vi "GetParam.vi"(8 "error in (no error)":errorcluster caption="entrée d'erreur (pas d'erreur)", 11 "Laplacian_kernel.lvclass":refnum<class "Laplacian_kernel.lvclass">) -> (0 "error out":errorcluster caption="sortie d'erreur", 2 "laplacian_kernel":cluster{"gamma":string}={"gamma"="None"}, 3 "Laplacian_kernel.lvclass":refnum<class "Laplacian_kernel.lvclass">)   [LabVIEW 2020, in "Laplacian_kernel.lvclass"]
doc: "Get Parameters"
uses:
  Laplacian_kernel.lvclass
  Laplacian_kernel.lvclass/Laplacian_kernel.ctl
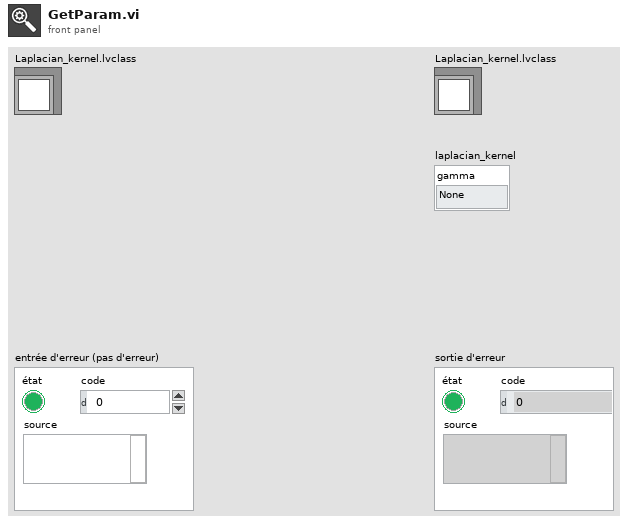
[diagram p1: front panel]
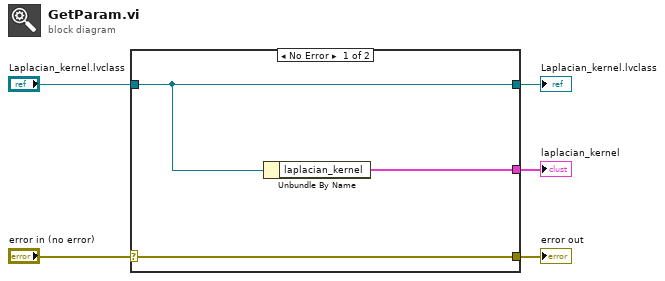
[diagram p0: block diagram]
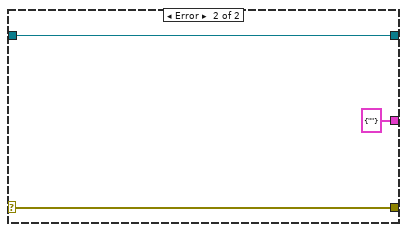
[diagram p2: hidden frame]
diagram:
  n1 = case shown="No Error" "error in (no error)" {
    selector: "error in (no error)" -> [w8 w10]
    tunnel: [w8 w10] -> w4
    tunnel: [w7 w11] -> w2
    tunnel: "Laplacian_kernel.lvclass" -> [w7 w11]
    tunnel: [w6 cluster{"gamma":string} {"gamma"=""} ("laplacian_kernel")] -> w1
    frame No Error {
      n2 = Unbundle By Name(w7) -> ("laplacian_kernel"=w6:cluster{"gamma":string})
    }
    frame Error {
    }
  }
  "error out" <- w4
  "Laplacian_kernel.lvclass" <- w2
  "laplacian_kernel" <- w1
